vi "DAQ_Static Dig Meas Configure and Measure.vi"(0 "DAQmx Task In":refnum<k21>, 11 "error in":errorcluster) -> (4 "DAQmx Task Out":refnum<k21>, 6 "Channel Line Identifiers":refnum<k21>[](array[refnum]), 8 "Line States":bool[](array[boolean]), 15 "error out":errorcluster)   [LabVIEW 2021, in "DAQ_Static Digital State Measurement.lvlib"]
doc: "Configure, initiate and fetch Static digital measurements from the channels configured."
uses:
  DAQ_Static Digital State Measurement.lvlib
  <vilib>/DAQmx/read.llb/DAQmx Read (Digital 1D Bool NChan 1Samp 1Line).vi
  <vilib>/DAQmx/miscellaneous.llb/DAQmx Fill In Error Info.vi
  <resource>/objmgr/daqmx.rc
panel:
  # "Outputs"
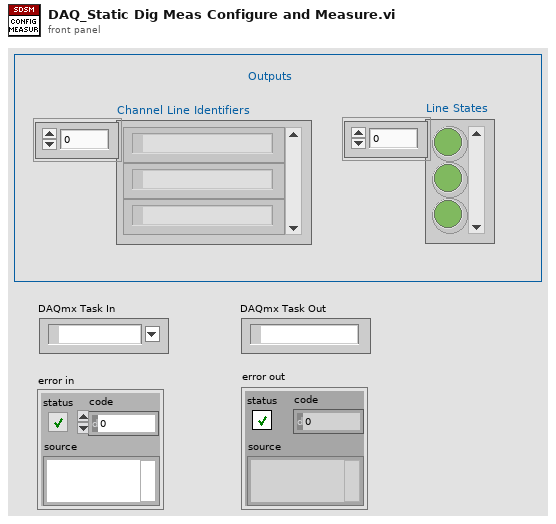
[diagram p1: front panel]
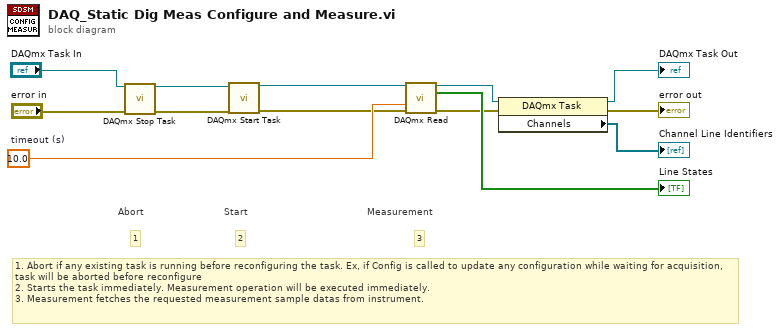
[diagram p0: block diagram]
diagram:
  w5 = 10.0  # timeout (s)
  # "2"
  # "Start"
  # "1"
  # "Abort"
  # "3"
  # "Measurement"
  # "1. Abort if any existing task is running before reconfiguring the task. Ex, if Config is called to update any configuration while waiting for acquisition, task will be aborted before reconfigure\n2. Starts the task immediately. Measurement operation will be executed immediately.\n3. Measurement fetches the requested measurement sample datas from instrument."
  n1 = call <vilib>:"DAQmx Stop Task.vi"("task/channels in"="DAQmx Task In", "error in"="error in") -> ("task out"=w7:refnum<k21>, "error out"=w6:errorcluster)  [unwired: 12 in]
  n2 = call <vilib>:"DAQmx Start Task.vi"("task/channels in"=w7, "error in"=w6) -> ("task out"=w4:refnum<k21>, "error out"=w3:errorcluster)  [unwired: 12 in]
  n3 = call-poly <vilib>:"DAQmx Read.vi"("task/channels in"=w4, "timeout"=w5, "error in"=w3) -> ("task out"=w1:refnum<k21>, "data"=→"Line States":bool[], "error out"=w2:errorcluster)  [unwired: 10 in]
  n4 = property class="DAQmx Task"(reference=w1, error in=w2) -> (reference out=→"DAQmx Task Out":refnum<k21>, error out=→"error out":errorcluster, "Channels"=→"Channel Line Identifiers":refnum<k21>[])
